vi "实验3-1.vi"() -> ()   [LabVIEW 2018]
panel:
  in  "停止":bool
  in  "开始":bool
  out "平均值":dbl
  out "最小值":dbl
  out "最大值":dbl
  out "波形图":dbl[](graph)
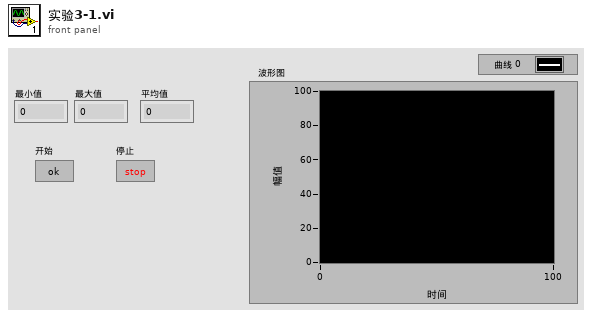
[diagram p1: front panel]
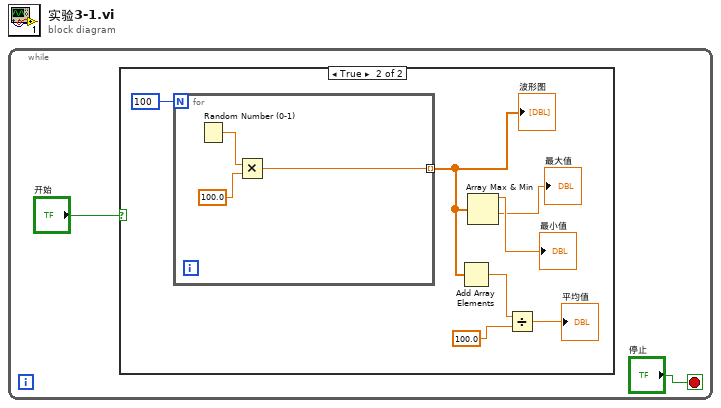
[diagram p0: block diagram]
diagram:
  n1 = while {
    stop <- "停止" stop-if-true
    n2 = case shown="True" "开始" {
      frame False {
      }
      frame True {
        n3 = for {
          N: 100 -> [_]
          tunnel: [w10] -> w6 mode=indexing
          n4 = Random Number (0-1)() -> (number: 0 to 1=w11:dbl)
          n5 = Multiply(x=w11, y=100.0) -> (x*y=w10:dbl)
        }
        "波形图" <- w6
        n6 = Add Array Elements(numeric array=w6) -> (sum=w5:dbl)
        n7 = Array Max & Min(array=w6) -> (max value=→"最小值":dbl, min value=→"最大值":dbl)  [unwired: 2 out]
        n8 = Divide(x=w5, y=100.0) -> (x/y=→"平均值":dbl)
      }
    }
  }
